vi "Write RFPM Session.vi"(8 "error in (no error)":errorcluster, 10 "RFPM Session":refnum<k15>, 11 "SA Path in":refnum<class "SA 18GHz Path.lvclass">) -> (0 "error out":errorcluster, 3 "SA Path out":refnum<class "SA 18GHz Path.lvclass">)   [LabVIEW 2023, in "RFFixtureCharact.RFPM.lvlib" / "SA 18GHz Path.lvclass"]
uses:
  SA 18GHz Path.lvclass
  SA 18GHz Path.lvclass/SA 18GHz Path.ctl
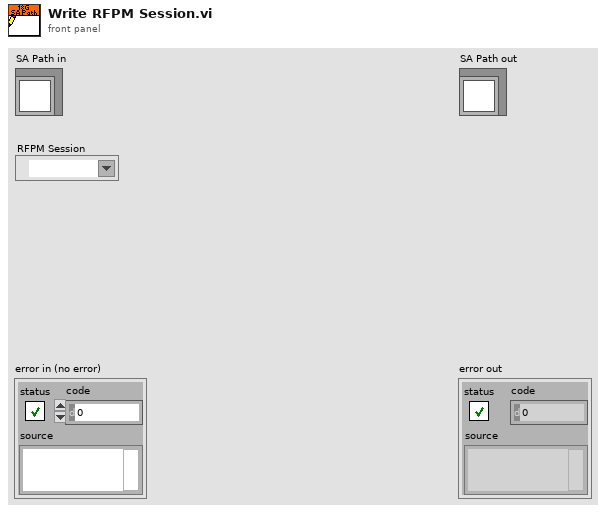
[diagram p1: front panel]
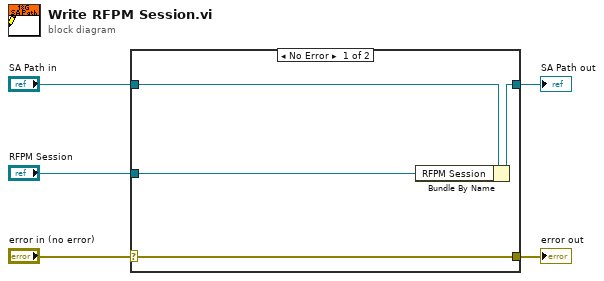
[diagram p0: block diagram]
diagram:
  n1 = case shown="No Error" "error in (no error)" {
    selector: "error in (no error)" -> [w9 w10]
    tunnel: [w9 w10] -> w4
    tunnel: [w7 w11] -> w2
    tunnel: "SA Path in" -> [w8 w11]
    tunnel: "RFPM Session" -> [w6 _]
    frame No Error {
      n2 = Bundle By Name(cluster=w8, "RFPM Session"=w6) -> (w7:refnum<class "SA 18GHz Path.lvclass">)
    }
    frame Error {
    }
  }
  "error out" <- w4
  "SA Path out" <- w2
